vi "Draw Markers.vi"(6 "Marker Options":T3={"Color"=16723218, "pen"={"Width"=2, "Style"=enum."Solid"}, "font"={"Font Name"="System Font", "Size"=16, "Strikeout?"=FALSE, "Italic?"=FALSE, "Underline?"=FALSE, "Outline?"=FALSE, "Shadow?"=FALSE, "Bold?"=FALSE, "FontColor"=6618880}, "caption"=""}, 8 "error in (no error)":errorcluster, 9 "Marker":T1={"Type"=enum."arrow", "X"=163.0, "Y"=1.0, "X2"=163.0, "Y2"=218.0, "Text"="Salam on Muhammad (SAW)"}, 10 "GrphChrt Refnum":refnum<vi>, 11 "picture":picture) -> (0 "error out":errorcluster, 3 "Picture out":picture)   [LabVIEW 2019]
doc: "Draw the appropriate line for markers, depending on the type"
uses:
  controls/MarkerOptions.ctl
  controls/MarkerInfo.ctl
  controls/markerType.ctl
  <vilib>/Utility/miscctls.llb/LVPoint32TypeDef.ctl
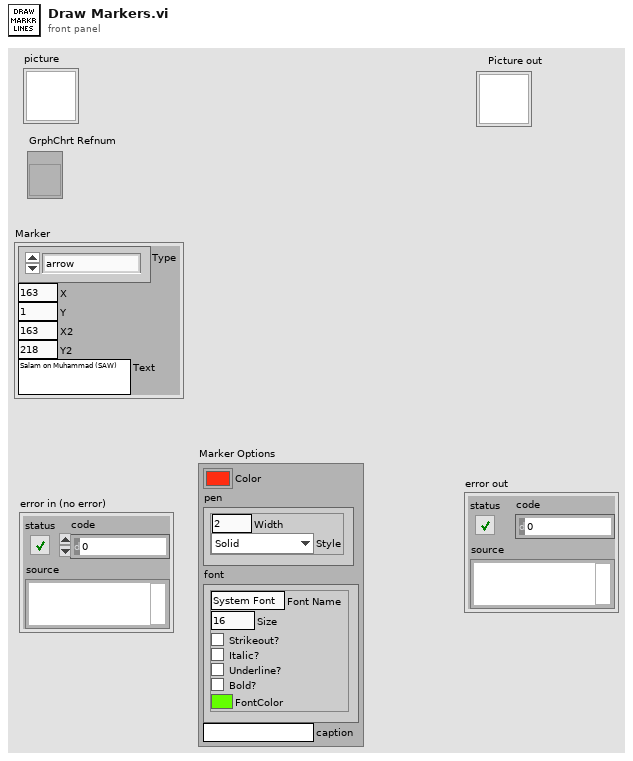
[diagram p1: front panel]
types:
  T1 = typedef "MarkerInfo.ctl" = cluster{"Type":T2, "X":dbl, "Y":dbl, "X2":dbl, "Y2":dbl, "Text":string}
  T2 = typedef "markerType.ctl" = enum16{"point", "arrow", "horiz", "vert", "vert range", "horiz range", "box"}
  T3 = typedef "MarkerOptions.ctl" = cluster{"Color":u32, "pen":cluster{"Width":u16, "Style":enum32{"Solid", "Dash", "Dot", "DashDot", "DashDotDot"}}, "font":cluster{"Font Name":string, "Size":i16, "Strikeout?":bool, "Italic?":bool, "Underline?":bool, "Outline?":bool, "Shadow?":bool, "Bold?":bool, "FontColor":u32}, "caption":string}
  T4 = typedef "LVPoint32TypeDef.ctl" = cluster{"Horizental":i32, "Vertical":i32}
  T5 = enum16{"User-specified Font", "Application Font", "System Font", "Dialog Font"}
  T6 = cluster{"Font Name:":string, "Size":i16, "Strikeout?":bool, "Italic?":bool, "Underline?":bool, "Outline?":bool, "Shadow?":bool, "Bold?":bool}
  T7 = typedef "LVRectTypeDef.ctl" = cluster{"Left":i16, "Top":i16, "Right":i16, "Bottom":i16}
  T8 = cluster{"Width":u16, "Style":enum32{"Solid", "Dash", "Dot", "DashDot", "DashDotDot"}}
  T9 = cluster{"Font Name":string, "Size":i16, "Strikeout?":bool, "Italic?":bool, "Underline?":bool, "Outline?":bool, "Shadow?":bool, "Bold?":bool, "FontColor":u32}
  T10 = cluster{"left":i16, "top":i16, "right":i16, "bottom":i16}
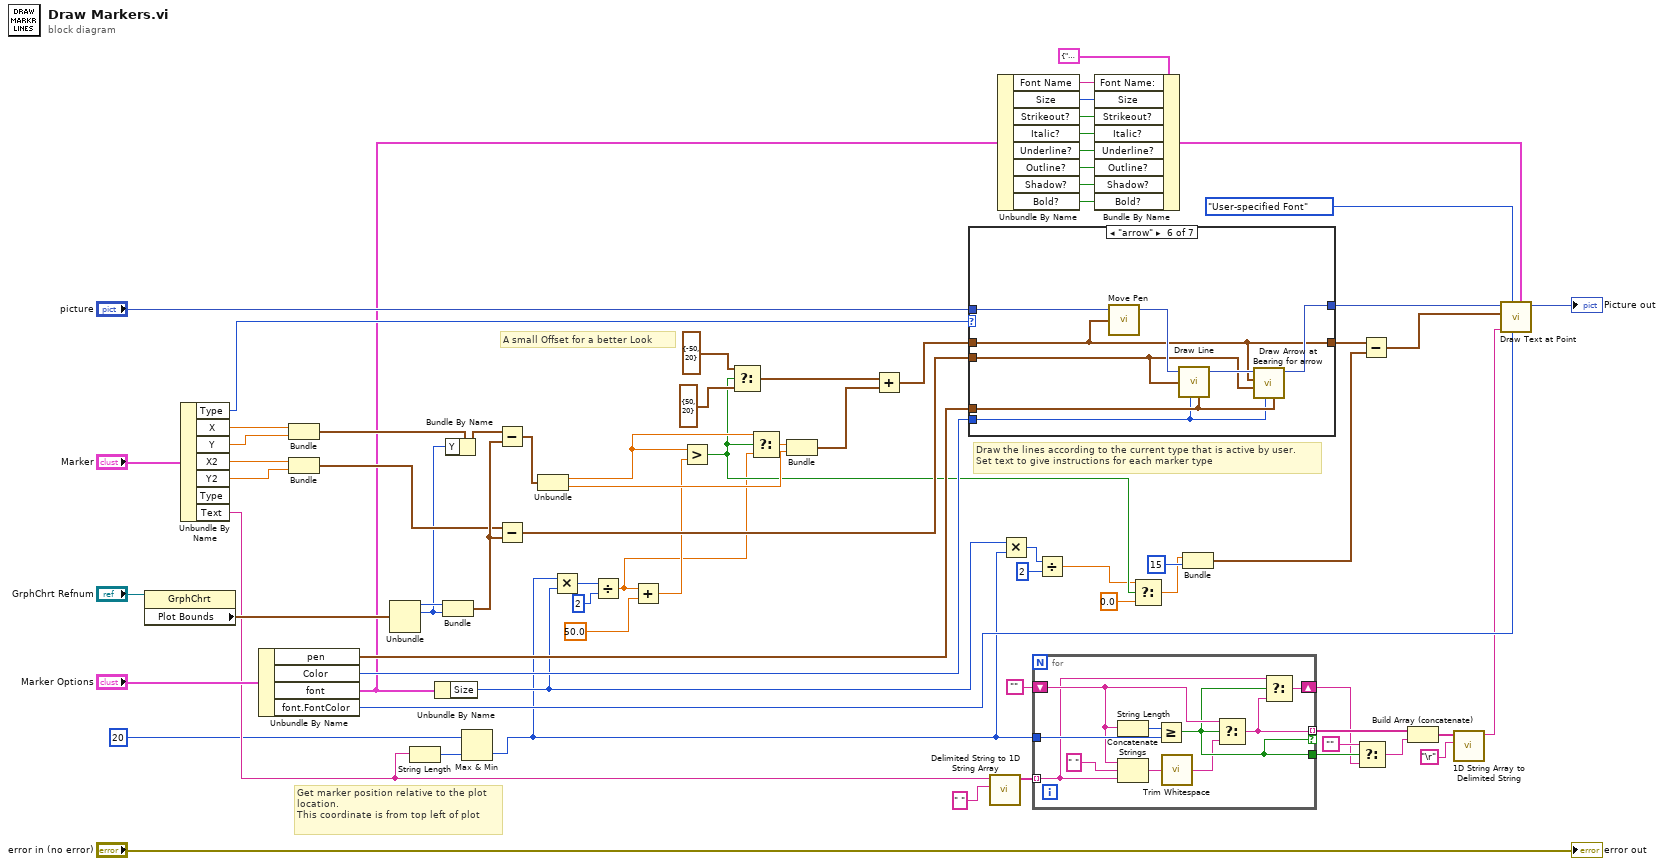
[diagram p0: block diagram]
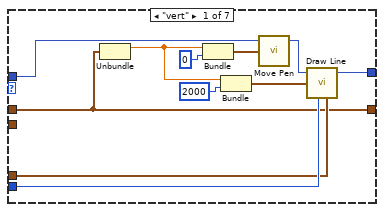
[diagram p2: hidden frame]
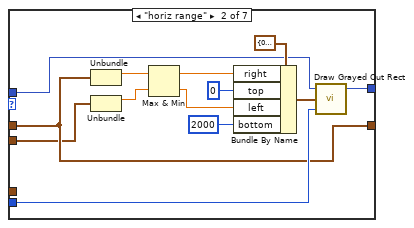
[diagram p3: hidden frame]
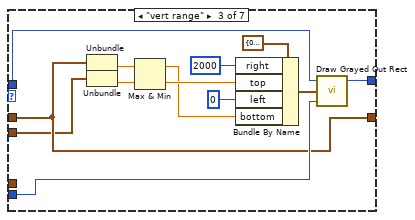
[diagram p4: hidden frame]
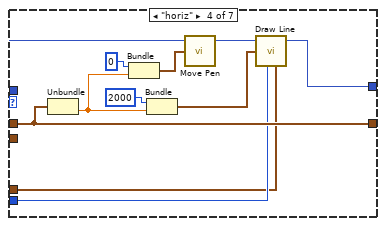
[diagram p5: hidden frame]
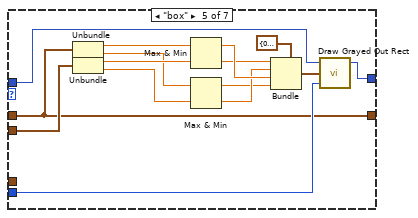
[diagram p6: hidden frame]
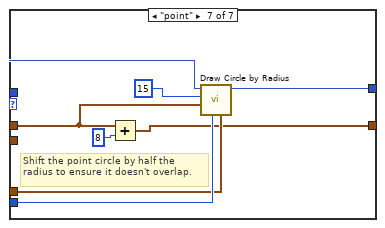
[diagram p7: hidden frame]
diagram:
  # "A small Offset for a better Look"
  # "Get marker position relative to the plot location.\nThis coordinate is from top left of plot"
  # "Draw the lines according to the current type that is active by user.\nSet text to give instructions for each marker type"
  n1 = property on="Property Node" class="GrphChrt"(reference="GrphChrt Refnum") -> ("Plot Bounds"=w54:T7)  [unwired: 1 in, 2 out]
  n2 = Unbundle By Name("Marker") -> ("Type"=w29:T2, "X"=w73:dbl, "Y"=w72:dbl, "X2"=w70:dbl, "Y2"=w69:dbl, "Text"=w6:string)  [unwired: 1 out]
  n3 = Unbundle By Name("Marker Options") -> ("pen"=w28:T8, "Color"=w27:u32, "font"=w26:T9, "font.FontColor"=w67:u32)
  n4 = Bundle("X"=w73, "Y"=w72) -> (w48:cluster{"X":dbl, "Y":dbl})  [unwired: 1 in]
  n5 = Bundle("X2"=w70, "Y2"=w69) -> (w49:cluster{"X2":dbl, "Y2":dbl})  [unwired: 1 in]
  n6 = Unbundle(w54) -> ("Left"=w55:i16, "Top"=w47:i16)  [unwired: 2 out]
  n7 = String Length(string=w6) -> (length=w4:i32)
  n8 = Unbundle By Name(w26) -> ("Size"=w7:i16)
  n9 = Bundle("Left"=w55, "Top"=w47) -> (w53:cluster{"Left":i16, "Top":i16})  [unwired: 1 in]
  n10 = Bundle By Name(cluster=w48, "Y"=w47) -> (w46:cluster{"X":dbl, "Y":dbl})
  n11 = Max & Min(x=20 ("y"), y=w4) -> (min(x,y)=w3:i32)  [unwired: 1 out]
  n12 = Subtract(x=w46, y=w53) -> (x-y=w23:cluster{dbl, dbl})
  n13 = Subtract(x=w49, y=w53) -> (x-y=w52:cluster{dbl, dbl})
  n14 = Unbundle(w23) -> (w20:dbl, w25:dbl)
  n15 = Multiply(x=w3, y=w7) -> (x*y=w8:i32)
  n16 = Divide(x=w8, y=2) -> (x/y=w2:dbl)
  n17 = Add(x=w2, y=50.0) -> (x+y=w11:dbl)
  n18 = Greater?(x=w20, y=w11) -> (0:w13:bool)
  n19 = Select(t=T4 {"Horizental"=-50, "Vertical"=20} ("y"), s=w13, f=T4 {"Horizental"=50, "Vertical"=20} ("y")) -> (s? t:f=w12:T4)
  n20 = Select(t=w20, s=w13, f=w2) -> (s? t:f=w17:dbl)
  n21 = Bundle(w17, w25) -> (w22:cluster{dbl, dbl})  [unwired: 1 in]
  n22 = Add(x=w12, y=w22) -> (x+y=w21:cluster{dbl, dbl})
  n23 = case shown="\"arrow\"" w29 {
    tunnel: w21 -> [w76 w97 w110 w116 w124 w139 w149]
    tunnel: [w84 w99 w112 w122 w136 w143 w154] -> w68
    tunnel: "picture" -> [w79 w91 w106 w113 w138 w145 w150]
    tunnel: w27 -> [w78 w98 w111 w115 w137 w141 w153]
    tunnel: w28 -> [w77 _ _ w114 _ w142 w151]
    tunnel: [w76 w97 w110 w116 w124 w139 w147] -> w56
    tunnel: w52 -> [_ w92 w107 _ w133 w140 _]
    frame "vert" {
      n24 = Unbundle(w76) -> (w86:dbl)  [unwired: 1 out]
      n25 = Bundle(w86, "top"=i16 0) -> (w80:cluster{dbl, "top":i16})  [unwired: 1 in]
      n26 = Bundle(w86, "top"=i16 2000) -> (w85:cluster{dbl, "top":i16})  [unwired: 1 in]
      n27 = call <vilib>:"Move Pen.vi"("new position"=w80, "picture"=w79) -> ("new picture"=w83:picture)  [unwired: 3 in]
      n28 = call <vilib>:"Draw Line.vi"("picture"=w83, "end point"=w85, "color(black)"=w78, "pen"=w77) -> ("new picture"=w84:picture)  [unwired: 5 in]
    }
    frame "horiz range" {
      n29 = Unbundle(w97) -> (w90:dbl)  [unwired: 1 out]
      n30 = Unbundle(w92) -> (w89:dbl)  [unwired: 1 out]
      n31 = Max & Min(x=w90, y=w89) -> (max(x,y)=w87:dbl, min(x,y)=w88:dbl)
      n32 = Bundle By Name(cluster=T10 {"left"=0, "top"=0, "right"=0, "bottom"=0} ("rect"), "right"=w87, "top"=i16 0, "left"=w88, "bottom"=i16 2000) -> (w95:T10)
      n33 = call <vilib>:"Draw Grayed Out Rect.vi"("color(black)"=w98, "rect"=w95, "picture"=w91) -> ("new picture"=w99:picture)  [unwired: 2 in]
    }
    frame "vert range" {
      n34 = Unbundle(w110) -> (w105:dbl)  [unwired: 1 out]
      n35 = Unbundle(w107) -> (w104:dbl)  [unwired: 1 out]
      n36 = Max & Min(x=w105, y=w104) -> (max(x,y)=w100:dbl, min(x,y)=w101:dbl)
      n37 = Bundle By Name(cluster=T10 {"left"=0, "top"=0, "right"=0, "bottom"=0} ("rect"), "right"=i16 2000 ("top"), "top"=w101, "left"=i16 0 ("bottom"), "bottom"=w100) -> (w108:T10)
      n38 = call <vilib>:"Draw Grayed Out Rect.vi"("color(black)"=w111, "rect"=w108, "picture"=w106) -> ("new picture"=w112:picture)  [unwired: 2 in]
    }
    frame "horiz" {
      n39 = Unbundle(w116) -> (w118:dbl)  [unwired: 1 out]
      n40 = Bundle("top"=i16 0, w118) -> (w120:cluster{"top":i16, dbl})  [unwired: 1 in]
      n41 = Bundle("top"=i16 2000, w118) -> (w123:cluster{"top":i16, dbl})  [unwired: 1 in]
      n42 = call <vilib>:"Move Pen.vi"("new position"=w120, "picture"=w113) -> ("new picture"=w121:picture)  [unwired: 3 in]
      n43 = call <vilib>:"Draw Line.vi"("picture"=w121, "end point"=w123, "color(black)"=w115, "pen"=w114) -> ("new picture"=w122:picture)  [unwired: 5 in]
    }
    frame "box" {
      n44 = Unbundle(w124) -> (w132:dbl, w128:dbl)
      n45 = Unbundle(w133) -> (w131:dbl, w127:dbl)
      n46 = Max & Min(x=w132, y=w131) -> (max(x,y)=w130:dbl, min(x,y)=w129:dbl)
      n47 = Max & Min(x=w128, y=w127) -> (max(x,y)=w125:dbl, min(x,y)=w126:dbl)
      n48 = Bundle(cluster=T10 {"left"=0, "top"=0, "right"=0, "bottom"=0} ("rect"), "left"=w129, "top"=w126, "right"=w130, "bottom"=w125) -> (w135:T10)
      n49 = call <vilib>:"Draw Grayed Out Rect.vi"("color(black)"=w137, "rect"=w135, "picture"=w138) -> ("new picture"=w136:picture)  [unwired: 2 in]
    }
    frame "arrow" {
      n50 = call <vilib>:"Move Pen.vi"("new position"=w139, "picture"=w145) -> ("new picture"=w146:picture)  [unwired: 3 in]
      n51 = call <vilib>:"Draw Line.vi"("picture"=w146, "end point"=w140, "color(black)"=w141, "pen"=w142) -> ("new picture"=w144:picture)  [unwired: 5 in]
      n52 = call "Draw Arrow at Bearing for arrow.vi"("pen"=w142, "color(black)"=w141, "P2"=w140, "P1"=w139, "new picture in"=w144) -> ("new picture out"=w143:picture)  [unwired: 6 in]
    }
    frame "point" {
      # "Shift the point circle by half the radius to ensure it doesn't overlap."
      n53 = Add(x=w149, y=8 ("Horizontal")) -> (x+y=w147:cluster{dbl, dbl})
      n54 = call <vilib>:"Draw Circle by Radius.vi"("pen"=w151, "color(black)"=w153, "pixel center"=w149, "radius"=i16 15, "picture"=w150) -> ("new picture"=w154:picture)  [unwired: 6 in]
    }
  }
  n55 = call <vilib>:"Delimited String to 1D String Array.vi"("delimiter"=" ", "delimited string"=w6) -> ("string array"=w38:string[])  [unwired: 9 in]
  n56 = Unbundle By Name(w26) -> ("Font Name"=w65:string, "Size"=w64:i16, "Strikeout?"=w63:bool, "Italic?"=w62:bool, "Underline?"=w61:bool, "Outline?"=w60:bool, "Shadow?"=w59:bool, "Bold?"=w58:bool)
  n57 = Multiply(x=w7, y=w3) -> (x*y=w9:i32)
  n58 = for {
    tunnel: w38 -> [w156] mode=indexing
    shift-right: [w159] -> w40
    shift-left: "" -> [w161]
    tunnel: w3 -> [w162]
    tunnel: [w160] -> w41 mode=indexing if=w157
    tunnel: [w157] -> w42
    n59 = String Length(string=w161) -> (length=w164:i32)
    n60 = Concatenate Strings(w161, " " ("string"), w156) -> (w158:string)
    n61 = Greater Or Equal?(x=w164, y=w162) -> (x >= y?=w157:bool)
    n62 = call <vilib>:"Trim Whitespace.vi"("string"=w158) -> ("trimmed string"=w155:string)  [unwired: 1 in]
    n63 = Select(t=w161, s=w157, f=w155) -> (s? t:f=w160:string)
    n64 = Select(t=w156, s=w157, f=w160) -> (s? t:f=w159:string)
  }
  n65 = Divide(x=w9, y=2) -> (x/y=w1:dbl)
  n66 = Bundle By Name(cluster=T6 {"Font Name:"="", "Size"=12, "Strikeout?"=FALSE, "Italic?"=FALSE, "Underline?"=FALSE, "Outline?"=FALSE, "Shadow?"=FALSE, "Bold?"=FALSE} ("[user-specified font]"), "Font Name:"=w65, "Size"=w64, "Strikeout?"=w63, "Italic?"=w62, "Underline?"=w61, "Outline?"=w60, "Shadow?"=w59, "Bold?"=w58) -> (w57:T6)
  n67 = Select(t=w1, s=w13, f=0.0) -> (s? t:f=w18:dbl)
  n68 = Bundle("f"=w18, "Vertical"=15) -> (w35:cluster{"f":dbl, "Vertical":i32})  [unwired: 1 in]
  n69 = Select(t="", s=w42, f=w40) -> (s? t:f=w44:string)
  n70 = Subtract(x=w56, y=w35) -> (x-y=w24:cluster{dbl, dbl})
  n71 = Build Array (concatenate)(w41, w44) -> (w33:string[])
  n72 = call <vilib>:"1D String Array to Delimited String.vi"("delimiter"="\r", "string array"=w33) -> ("delimited string"=w31:string)  [unwired: 9 in]
  n73 = call <vilib>:"Draw Text at Point.vi"("[user-specified font]"=w57, "text color(black)"=w67, "desired font(Application)"=T5."User-specified Font", "text"=w31, "origin"=w24, "picture"=w68) -> ("new picture"=→"Picture out":picture)  [unwired: 4 in, 1 out]
  "error out" <- "error in (no error)"
